vi "Force-processing-stop.vi"(8 "error in":errorcluster, 11 "Data ref. in":refnum<data-value>) -> (0 "error IO":errorcluster, 3 "Data ref.":refnum<data-value>)   [LabVIEW 2013, in "CameraVision.lvlib" / "CV-Main.lvclass"]
uses:
  CV-Main.lvclass
  CV-Main.lvclass/CV-Main.ctl
  Read Processing.vi
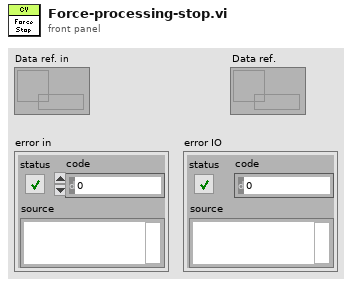
[diagram p1: front panel]
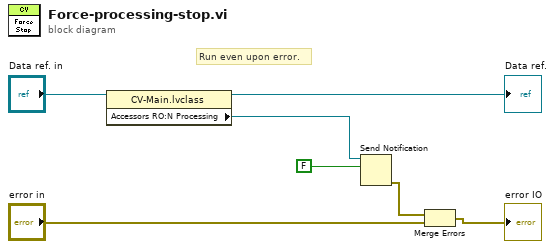
[diagram p0: block diagram]
diagram:
  # "Run even upon error."
  n1 = property class="CV-Main.lvclass"(reference="Data ref. in") -> (reference out=→"Data ref.":refnum<data-value>, "Accessors RO:N Processing"=w1:refnum<notifier>)  [unwired: 1 in, 1 out]
  n2 = Send Notification(notification=FALSE, notifier=w1) -> (error out=w2:errorcluster)  [unwired: 1 in, 1 out]
  n3 = Merge Errors(w2, "error in") -> (→"error IO":errorcluster)
